vi "Unlock.vi"(8 "error in (no error)":errorcluster, 11 "B&K In":refnum<class "B&K Precision 9120 series.lvclass">) -> (0 "error out":errorcluster, 3 "B&K Out":refnum<class "B&K Precision 9120 series.lvclass">)   [LabVIEW 2014, in "B&K Precision 9120 series.lvclass"]
uses:
  B&K Precision 9120 series.lvclass
  B&K Precision 9120 series.lvclass/B&K Precision 9120 series.ctl
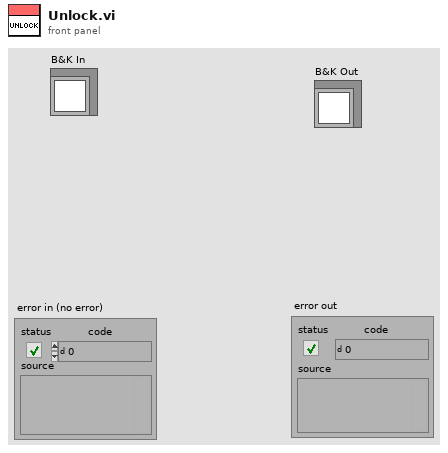
[diagram p1: front panel]
types:
  T1 = typedef "Semaphore RefNum" = refnum<k1>
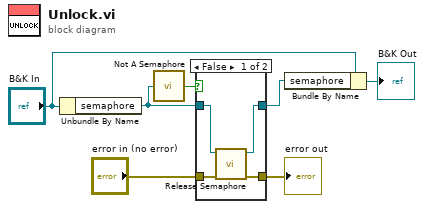
[diagram p0: block diagram]
diagram:
  n1 = Unbundle By Name("B&K In") -> ("semaphore"=w4:T1)
  n2 = call <vilib>:"Not A Semaphore.vi"("semaphore"=w4) -> ("not a semaphore"=w5:bool)
  n3 = case shown="False" w5 {
    tunnel: [w8 w12] -> w2
    tunnel: w4 -> [w11 w12]
    tunnel: "error in (no error)" -> [w10 w13]
    tunnel: [w9 w13] -> w1
    frame False {
      n4 = call <vilib>:"Release Semaphore.vi"("error in (no error)"=w10, "semaphore"=w11) -> ("error out"=w9:errorcluster, "semaphore out"=w8:T1)  [unwired: 4 in]
    }
    frame True {
    }
  }
  "error out" <- w1
  n5 = Bundle By Name(cluster="B&K In", "semaphore"=w2) -> (→"B&K Out":refnum<class "B&K Precision 9120 series.lvclass">)
